vi "Queue Comms DeQueue.vi"(8 "error in":errorcluster) -> (0 "error out":errorcluster, 2 "element":T1)   [LabVIEW 2018, in "Database.lvlib"]
uses:
  Database.lvlib
  Private Controls/Module Data Cluster.ctl
  Private Controls/Module Action.ctl
  Private Controls/Queue FG Action.ctl
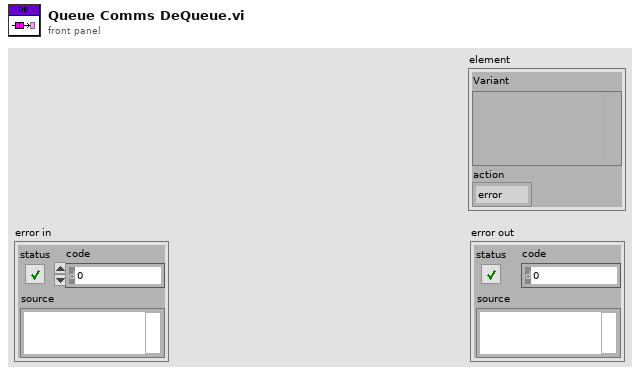
[diagram p1: front panel]
types:
  T1 = typedef "Database.lvlib/Module Data Cluster.ctl" = cluster{"Variant":variant, "action":T2}
  T2 = typedef "Database.lvlib/Module Action.ctl" = enum16{"error", "exit", "init", "Read Database Record", "Query Timing", "Update record", "Insert Record", "Release Connection"}
  T3 = typedef "Database.lvlib/Queue FG Action.ctl" = enum16{"Release", "Get", "Set"}
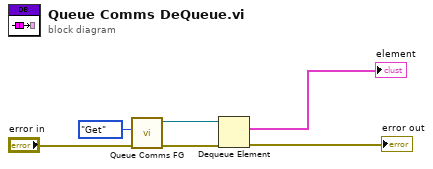
[diagram p0: block diagram]
diagram:
  n1 = call "Queue Comms FG.vi"("error in"="error in", "Action"=Queue_FG_Action."Get") -> ("error out"=w6:errorcluster, "queue out"=w5:refnum<queue>)  [unwired: 8 in]
  n2 = Dequeue Element(queue=w5, error in (no error)=w6) -> (element=→"element":T1, error out=→"error out":errorcluster)  [unwired: 1 in, 2 out]
